vi "get_z_intensity_tuples_memory_size.vi"(8 "error in (no error)":errorcluster, 11 "FPGAWrapperAK101022Resonance in":refnum<class "FPGAWrapperAK101022Resonance.lvclass">) -> (0 "error out":errorcluster, 2 "z/intensity memory size":i32, 3 "FPGAWrapperAK101022Resonance out":refnum<class "FPGAWrapperAK101022Resonance.lvclass">)   [LabVIEW 2010, in "FPGAWrapperAK101022Resonance.lvclass"]
uses:
  FPGAWrapperAK101022Resonance.lvclass
  FPGAWrapperAK101022Resonance.lvclass/FPGAWrapperAK101022Resonance.ctl
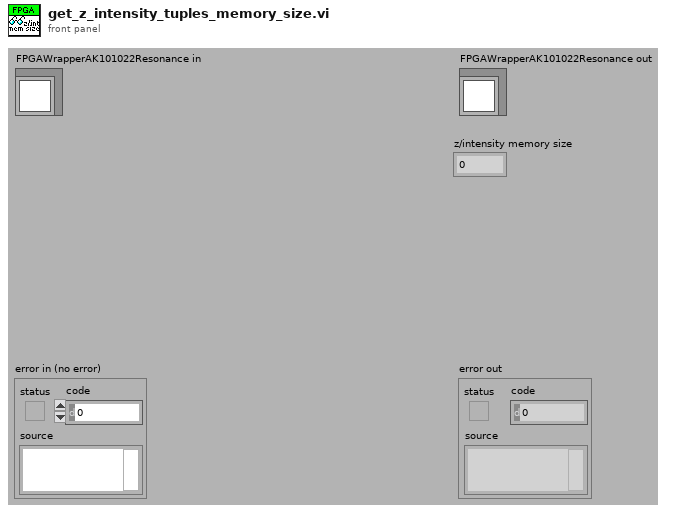
[diagram p1: front panel]
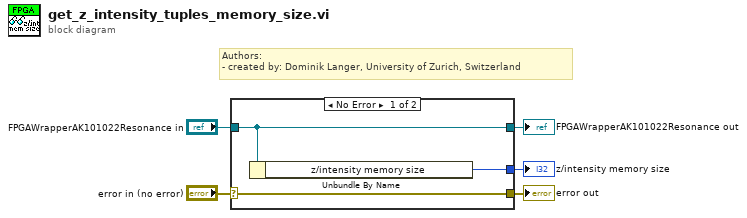
[diagram p0: block diagram]
diagram:
  # "Authors: \n- created by: Dominik Langer, University of Zurich, Switzerland"
  n1 = case shown="No Error" "error in (no error)" {
    selector: "error in (no error)" -> [w8 w10]
    tunnel: [w8 w10] -> w4
    tunnel: [w7 w9] -> w2
    tunnel: "FPGAWrapperAK101022Resonance in" -> [w7 w9]
    tunnel: [w6 _] -> w1
    frame No Error {
      n2 = Unbundle By Name(w7) -> ("z/intensity memory size"=w6:i32)
    }
    frame Error {
    }
  }
  "error out" <- w4
  "FPGAWrapperAK101022Resonance out" <- w2
  "z/intensity memory size" <- w1
